vi "ConstructImageSavePath.vi"(9 "Y Position":dbl, 10 "X Position":dbl, 11 "Time Stamp":string) -> (3 "appended path":path)   [LabVIEW 2024]
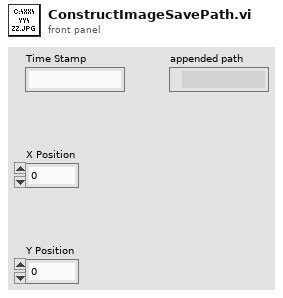
[diagram p1: front panel]
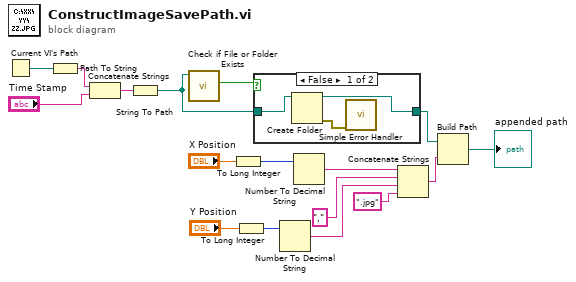
[diagram p0: block diagram]
diagram:
  n1 = Current VI's Path() -> (path=w12:path)
  n2 = Path To String(path=w12) -> (string=w11:string)
  n3 = Concatenate Strings(w11, "Time Stamp") -> (w10:string)
  n4 = String To Path(string=w10) -> (path=w14:path)
  n5 = call <vilib>:"Check if File or Folder Exists.vi"("path"=w14) -> ("file or folder exists?"=w13:bool)  [unwired: 8 in, 2 out]
  n6 = To Long Integer(number="X Position") -> (32bit integer=w2:i32)
  n7 = To Long Integer(number="Y Position") -> (32bit integer=w3:i32)
  n8 = case shown="False" w13 {
    tunnel: w14 -> [w20 w21]
    tunnel: [w19 w21] -> w15
    frame False {
      n9 = Create Folder(path (use dialog)=w20) -> (created path=w19:path, error out=w18:errorcluster)  [unwired: 2 in, 1 out]
      n10 = call <vilib>:"Simple Error Handler.vi"("error in (no error)"=w18) -> ()  [unwired: 4 in, 5 out]
    }
    frame True {
    }
  }
  n11 = Number To Decimal String(number=w3) -> (decimal integer string=w8:string)  [unwired: 1 in]
  n12 = Number To Decimal String(number=w2) -> (decimal integer string=w6:string)  [unwired: 1 in]
  n13 = Concatenate Strings(w6, "," ("string"), w8, ".jpg" ("string")) -> (w5:string)
  n14 = Build Path(base path=w15, name or relative path=w5) -> (appended path=→"appended path":path)
